vi "PRIME Detector Send Offsets.vi"(8 "error in (no error)":errorcluster, 10 "Offsets":u16[][](array[numeric])=[[0, 0, 0, 0, 0, 0, 0, 0, 0, 0, 0, 0, 0, 0, 0, 0, 0, 0, 0, 0, 0, 0, 0, 0, 0, 0, 0, 0, 0, 0, 0, 0]] format="%04x", 11 "connection ID":refnum<k5>) -> (0 "error out":errorcluster, 3 "connection ID out":refnum<k5>)   [LabVIEW 2024, in "PRIME Detector.lvclass"]
uses:
  PRIME Detector.lvclass
panel:
  out "Command":string
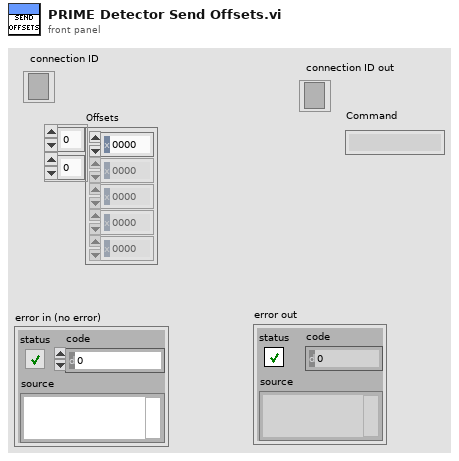
[diagram p1: front panel]
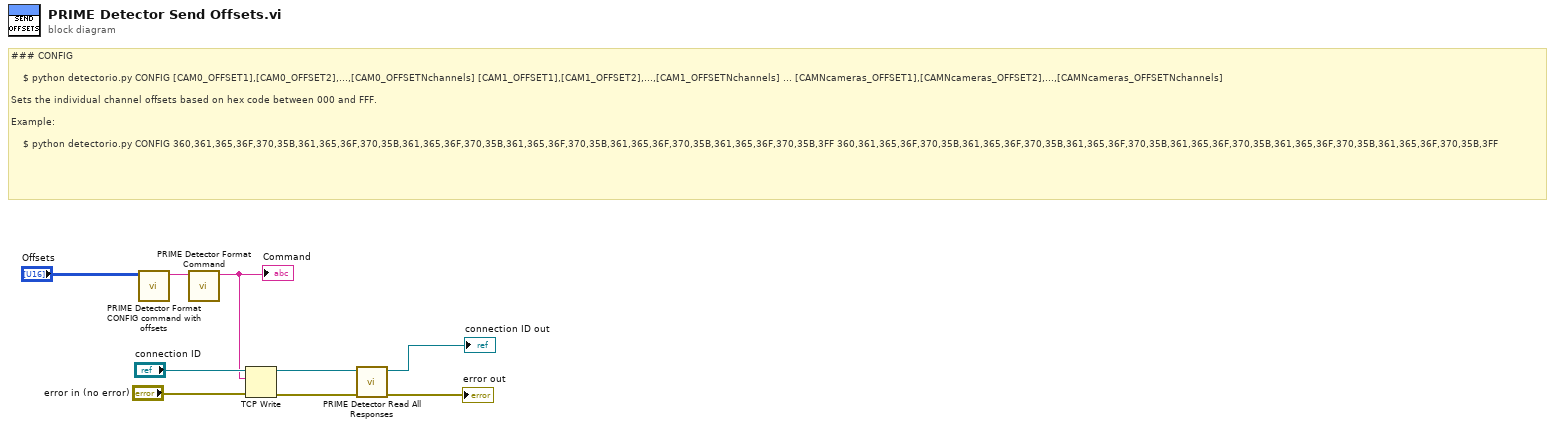
[diagram p0: block diagram]
diagram:
  # "### CONFIG\n\n    $ python detectorio.py CONFIG [CAM0_OFFSET1],[CAM0_OFFSET2],...,[CAM0_OFFSETNchannels] [CAM1_OFFSET1],[CAM1_OFFSET2],...,[CAM1_OFFSETNchannels] ... [CAMNcameras_OFFSET1],[CAMNcameras_OFFSET2],...,[CAMNcameras_OFFSETNchannels]\n\nSets the individual channel offsets based on hex code between 000 and FFF. \n\nExample:\n\n    $ python detectorio.py CONFIG 360,361,365,36F,370,35B,361,365,36F,370,35B,361,365,36F,370,35B,361,365,36F,370,35B,361,365,36F,370,35B,361,365,36F,370,35B,3FF 360,361,365,36F,370,35B,361,365,36F,370,35B,361,365,36F,370,35B,361,365,36F,370,35B,361,365,36F,370,35B,361,365,36F,370,35B,3FF"
  n1 = call "PRIME Detector Format CONFIG command with offsets.vi"("Offsets"="Offsets") -> ("Command"=w3:string)  [unwired: 10 in]
  n2 = call "PRIME Detector Format Command.vi"("Command"=w3) -> ("TCP String"=w2:string)  [unwired: 10 in]
  "Command" <- w2
  n3 = TCP Write(connection ID="connection ID", data in=w2, error in (no error)="error in (no error)") -> (connection ID out=w7:refnum<k5>, error out=w6:errorcluster)  [unwired: 1 in, 1 out]
  n4 = call "PRIME Detector Read All Responses.vi"("error in"=w6, "connection ID"=w7) -> ("error out"=→"error out":errorcluster, "connection ID out"=→"connection ID out":refnum<k5>)  [unwired: 6 in, 2 out]
